vi "createReportServerIDFrame.vi"(8 "error in (no error)":errorcluster, 9 "TriggerIRQ":bool, 10 "WaitForTrigger":bool, 11 "ILC in":refnum<class "ILC.lvclass">) -> (0 "error out":errorcluster, 2 "Frame":T1 {"Data" format="%02x"}, 3 "ILC out":refnum<class "ILC.lvclass">)   [LabVIEW 2015, in "RTILC.lvlib" / "ILC.lvclass"]
uses:
  ILC.lvclass
  Common_RT_Modbus/DataTypes/Frame.ctl
  Common_RT_Modbus/DynamicFrameBuilder/DynamicFrameBuilder.lvclass
  ILC.lvclass/ILC.ctl
  Common_RT_Modbus/RTModbus.lvlib
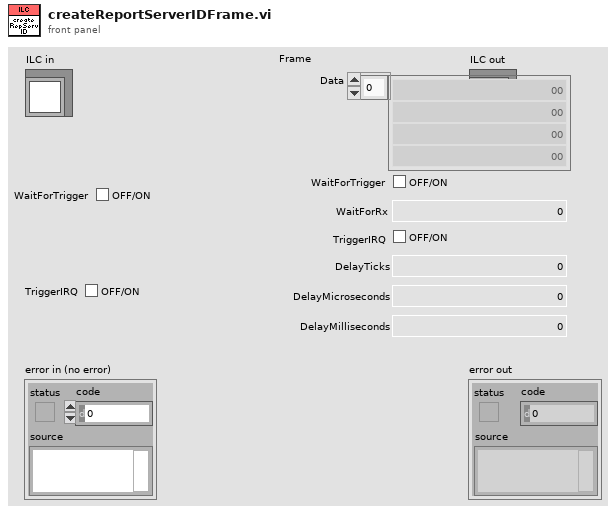
[diagram p1: front panel]
types:
  T1 = typedef "RTModbus.lvlib/Frame.ctl" = cluster{"Data":u8[], "WaitForTrigger":bool, "WaitForRx":u16, "TriggerIRQ":bool, "DelayTicks":u16, "DelayMicroseconds":u16, "DelayMilliseconds":u16}
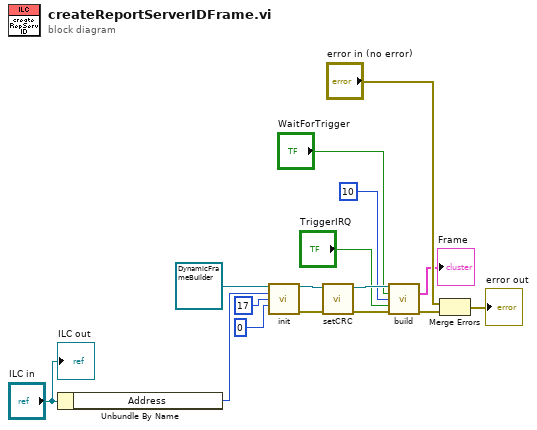
[diagram p0: block diagram]
diagram:
  n1 = Unbundle By Name("ILC in") -> ("Address"=w3:u8)
  n2 = call "init.vi"("DynamicFrameBuilder in"=refnum<class "DynamicFrameBuilder.lvclass"> refnum ("RTModbus.lvlib:DynamicFrameBuilder.lvclass"), "Address"=w3, "Function"=u8 17, "DataSize"=0) -> ("DynamicFrameBuilder out"=w12:refnum<class "DynamicFrameBuilder.lvclass">, "error out"=w9:errorcluster)  [unwired: 10 in]
  n3 = call "setCRC.vi"("error in (no error)"=w9, "DynamicFrameBuilder in"=w12) -> ("error out"=w8:errorcluster, "DynamicFrameBuilder out"=w11:refnum<class "DynamicFrameBuilder.lvclass">)  [unwired: 8 in]
  n4 = call "build.vi"("DynamicFrameBuilder in"=w11, "WaitForTrigger"="WaitForTrigger", "WaitForRxTimeout"=u16 10, "TriggerIRQ"="TriggerIRQ", "error in (no error)"=w8) -> ("Frame"=→"Frame":T1, "error out"=w7:errorcluster)  [unwired: 8 in, 1 out]
  n5 = Merge Errors("error in (no error)", w7) -> (→"error out":errorcluster)
  "ILC out" <- "ILC in"
